vi "CreateWorldAndBody.vi"(8 "error in (no error)":errorcluster, 9 "FieldSizeY":i32=15, 10 "FieldSizeX":i32=10, 11 "Snake in":refnum<class "Snake.lvclass">) -> (0 "error out":errorcluster, 3 "Snake out":refnum<class "Snake.lvclass">)   [LabVIEW 2014, in "Snake.lvclass"]
uses:
  Snake.lvclass
  Snake.lvclass/Snake.ctl
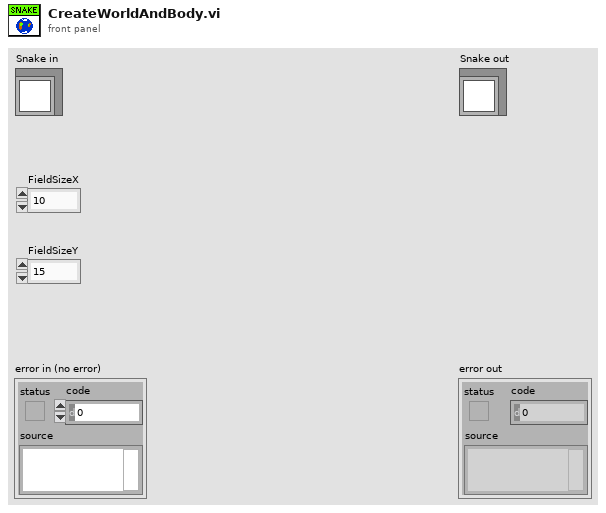
[diagram p1: front panel]
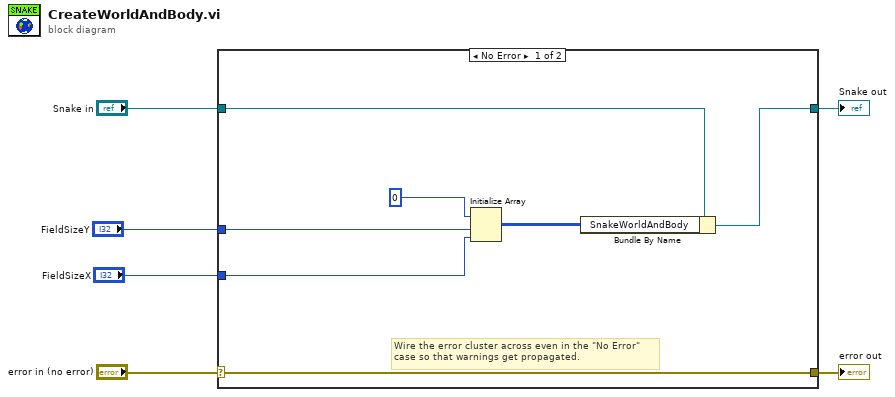
[diagram p0: block diagram]
diagram:
  n1 = case shown="No Error" "error in (no error)" {
    selector: "error in (no error)" -> [w13 w15]
    tunnel: [w13 w15] -> w5
    tunnel: [w8 w14] -> w3
    tunnel: "Snake in" -> [w9 w14]
    tunnel: "FieldSizeX" -> [w11 _]
    tunnel: "FieldSizeY" -> [w12 _]
    frame No Error {
      # "Wire the error cluster across even in the \"No Error\"\ncase so that warnings get propagated."
      n2 = Initialize Array(u32 0, w12, w11) -> (w7:u32[][])
      n3 = Bundle By Name(cluster=w9, "SnakeWorldAndBody"=w7) -> (w8:refnum<class "Snake.lvclass">)
    }
    frame Error {
    }
  }
  "error out" <- w5
  "Snake out" <- w3
